vi "string_to_boolean.vi"(8 "error in":errorcluster, 11 "string":string) -> (0 "error out":errorcluster, 3 "boolean":bool)   [LabVIEW 2013]
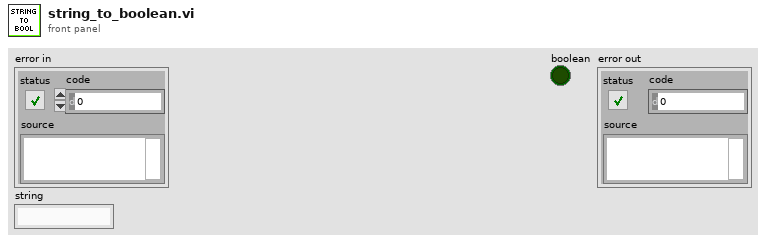
[diagram p1: front panel]
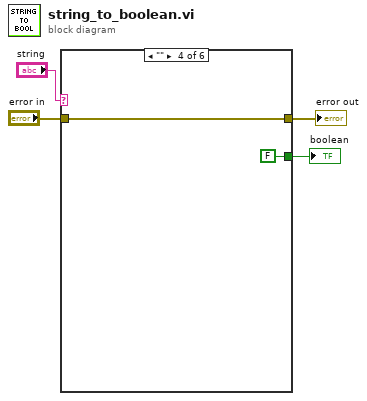
[diagram p0: block diagram]
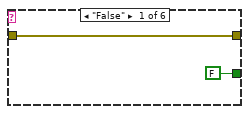
[diagram p2: hidden frame]
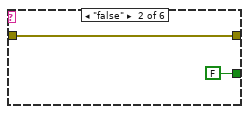
[diagram p3: hidden frame]
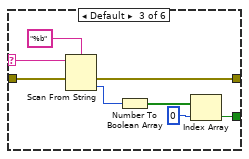
[diagram p4: hidden frame]
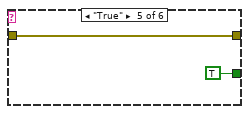
[diagram p5: hidden frame]
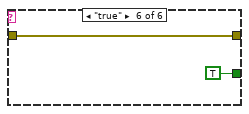
[diagram p6: hidden frame]
diagram:
  n1 = case shown="\"\"" "string" {
    selector: "string" -> [_ _ w11 _ _ _]
    tunnel: "error in" -> [w5 w7 w12 w17 w19 w21]
    tunnel: [FALSE FALSE w10 FALSE TRUE TRUE] -> w2
    tunnel: [w5 w7 w9 w17 w19 w21] -> w1
    frame "False" {
    }
    frame "false" {
    }
    frame Default {
      n2 = Scan From String(format string="%b", input string=w11, error in=w12) -> (error out=w9:errorcluster, output 1=w14:i32)  [unwired: 2 in, 2 out]
      n3 = Number To Boolean Array(number=w14) -> (Boolean array=w15:bool[])
      n4 = Index Array(array=w15, index=0) -> (element=w10:bool)
    }
    frame "" {
    }
    frame "True" {
    }
    frame "true" {
    }
  }
  "boolean" <- w2
  "error out" <- w1
